vi "gen_ref.vi"(8 "error in (no error)":errorcluster, 10 "Name":string="Trigger", 11 "reference":refnum<vi>) -> (0 "error out":errorcluster, 2 "Array":string[](array[string]), 3 "Ref":refnum<vi>)   [LabVIEW 2013]
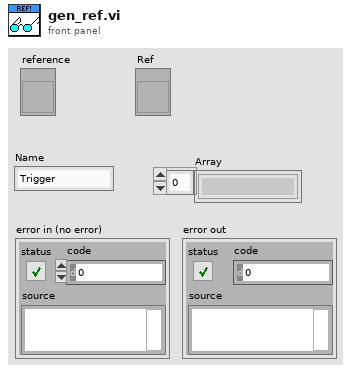
[diagram p1: front panel]
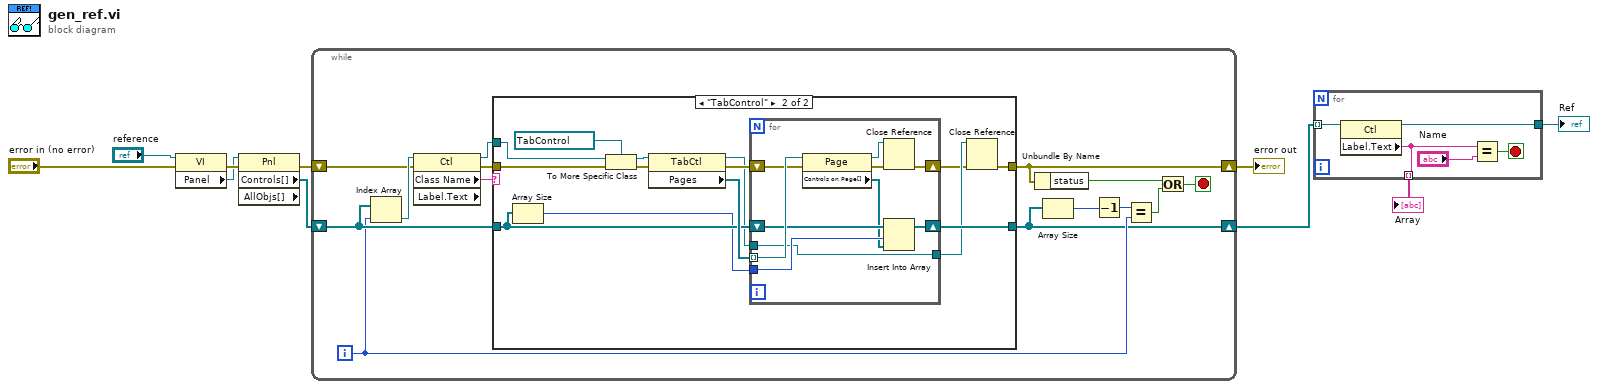
[diagram p0: block diagram]
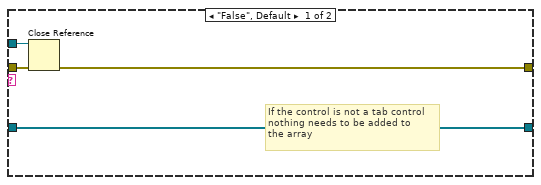
[diagram p2: hidden frame]
diagram:
  n1 = property class="VI"(reference="reference", error in="error in (no error)") -> (error out=w10:errorcluster, "Panel"=w9:refnum<vi>)  [unwired: 1 out]
  n2 = property class="Pnl" props=["Controls[]", "AllObjs[]"](reference=w9, error in=w10) -> (error out=w3:errorcluster, "Controls[]"=w7:refnum<vi>[])  [unwired: 2 out]
  n3 = while {
    shift-right: [w17] -> w6
    shift-left: w7 -> [w23]
    shift-right: [w14] -> w4
    shift-left: w3 -> [w16]
    i -> [w18]
    stop <- w12 stop-if-true
    n4 = Index Array(array=w23, index=w18) -> (element=w19:refnum<vi>)
    n5 = property class="Ctl" props=["Class Name", "Label", "Text"](reference=w19, error in=w16) -> (reference out=w24:refnum<vi>, error out=w15:errorcluster, "Class Name"=w22:string)  [unwired: 1 out]
    n6 = case shown="\"TabControl\"" w22 {
      tunnel: w24 -> [w27 w42]
      tunnel: w23 -> [w28 w38]
      tunnel: [w28 w39] -> w17
      tunnel: w15 -> [w26 w35]
      tunnel: [w25 w31] -> w14
      frame "False", Default {
        # "If the control is not a tab control\nnothing needs to be added to\nthe array"
        n7 = Close Reference(reference=w27, error in (no error)=w26) -> (error out=w25:errorcluster)
      }
      frame "TabControl" {
        n8 = Array Size(array=w38) -> (size(s)=w36:i32)
        n9 = To More Specific Class(target class=refnum<vi> refnum ("Tab Control"), reference=w42, error in=w35) -> (specific class reference=w41:refnum<vi>, error out=w34:errorcluster)
        n10 = property class="TabCtl"(reference=w41, error in=w34) -> (reference out=w32:refnum<vi>, error out=w33:errorcluster, "Pages"=w40:refnum<vi>[])
        n11 = for {
          tunnel: w40 -> [w52] mode=indexing
          tunnel: w36 -> [w50]
          shift-right: [w51] -> w39
          shift-left: w38 -> [w49]
          tunnel: w32 -> [w46]
          tunnel: [w46] -> w30
          shift-right: [w43] -> w29
          shift-left: w33 -> [w47]
          n12 = property class="Page"(reference=w52, error in=w47) -> (reference out=w45:refnum<vi>, error out=w44:errorcluster, "Controls on Page[]"=w48:refnum<vi>[])
          n13 = Close Reference(reference=w45, error in (no error)=w44) -> (error out=w43:errorcluster)
          n14 = Insert Into Array(array=w49, index=w50, new element=w48) -> (w51:refnum<vi>[])
        }
        n15 = Close Reference(reference=w30, error in (no error)=w29) -> (error out=w31:errorcluster)
      }
    }
    n16 = Unbundle By Name(w14) -> ("status"=w11:bool)
    n17 = Array Size(array=w17) -> (size(s)=w21:i32)
    n18 = Decrement(x=w21) -> (x-1=w20:i32)
    n19 = Equal?(x=w20, y=w18) -> (x = y?=w13:bool)
    n20 = Or(x=w11, y=w13) -> (x .or. y?=w12:bool)
  }
  "error out" <- w4
  n21 = for {
    tunnel: w6 -> [w57] mode=indexing
    tunnel: [w56] -> w8
    tunnel: [w53] -> w1 mode=indexing
    stop <- w55 stop-if-true
    n22 = property class="Ctl"(reference=w57) -> (reference out=w56:refnum<vi>, "Label.Text"=w53:string)  [unwired: 1 in, 1 out]
    n23 = Equal?(x=w53, y="Name") -> (x = y?=w55:bool)
  }
  "Ref" <- w8
  "Array" <- w1
